vi "Scan Engine Initialization VI.vi"(8 "error in (no error)":errorcluster, 10 "Custom XML":string, 11 "Device Item Ref in":T1 format="%.0x") -> (0 "error out":errorcluster, 3 "Device Item Ref out":T1 format="%.0x")   [LabVIEW 2016, in "Scan Engine Custom Device.lvlib"]
uses:
  Scan Engine Custom Device.lvlib
  <vilib>/NI Veristand/Custom Device API/Custom Device Item Ref.ctl
  <vilib>/NI Veristand/Custom Device API/Custom Device Channel.ctl
  <vilib>/NI Veristand/Custom Device API/Custom Device Channel Type.ctl
  Globals/Property Strings.vi
  <vilib>/NI Veristand/Custom Device API/Set Item Property (U16).vi
  <vilib>/NI Veristand/Custom Device API/Set Item Property (String).vi
  <vilib>/NI Veristand/Custom Device API/Custom Device API.lvlib
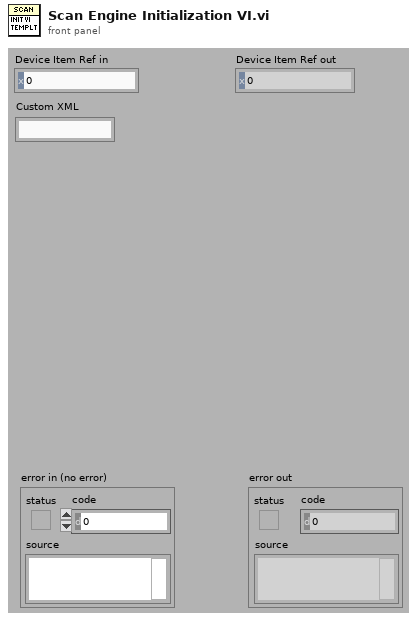
[diagram p1: front panel]
types:
  T1 = typedef "Custom Device API.lvlib/Custom Device Item Ref.ctl" = u64
  T2 = typedef "Custom Device API.lvlib/Custom Device Channel.ctl" = cluster{"Type":T3, "Units":string, "Default Value":dbl, "Faultable":bool, "Scalable":bool}
  T3 = typedef "Custom Device API.lvlib/Custom Device Channel Type.ctl" = enum16{"Input", "Output"}
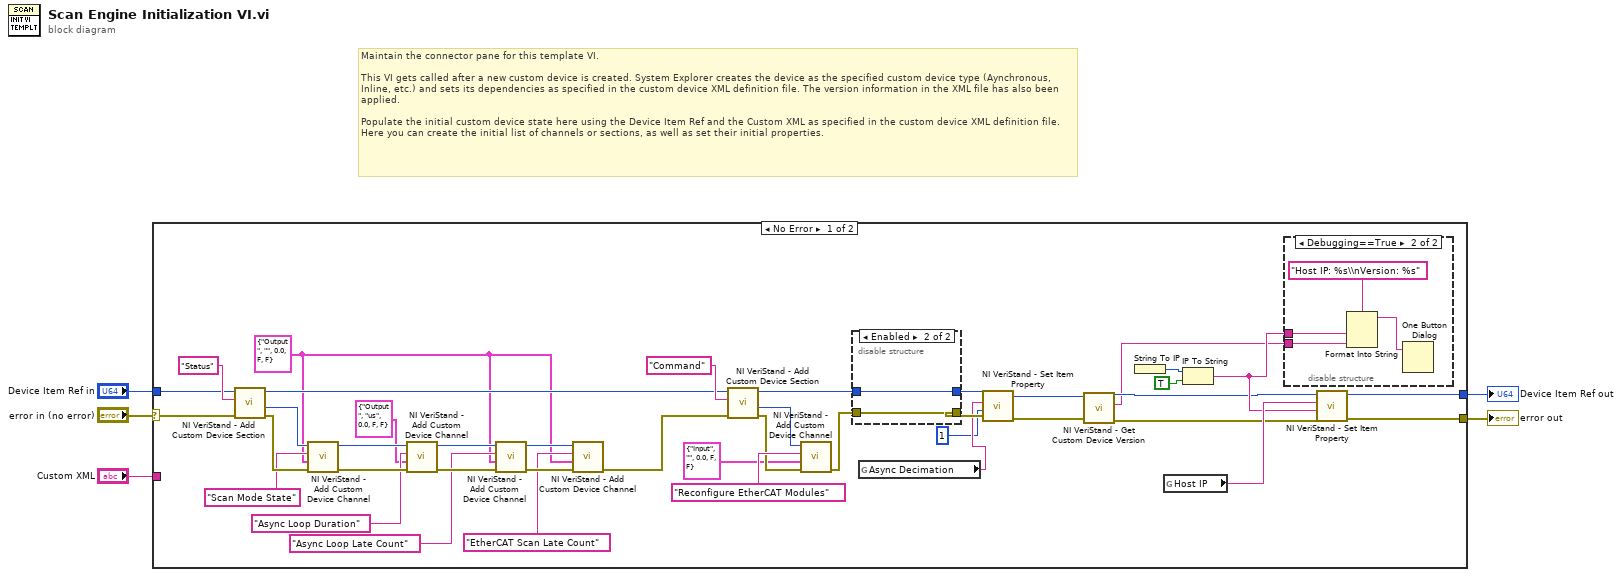
[diagram p0: block diagram]
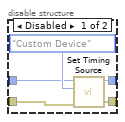
[diagram p3: hidden frame]
diagram:
  # "Maintain the connector pane for this template VI.\n\nThis VI gets called after a new custom device is created. System Explorer creates the device as the specified custom device type (Aynchronous, Inline, etc.) and sets its dependencies as specified in the custom device XML definition file. The version information in the XML file has also been applied.\n\nPopulate the initial custom device state here using the Device Item Ref and the Custom XML as specified in the custom device XML definition file. Here you can create the initial list of channels or sections, as well as set their initial properties."
  n1 = case shown="No Error" "error in (no error)" {
    selector: "error in (no error)" -> [w29 w59]
    tunnel: [w14 w59] -> w5
    tunnel: [w15 w58] -> w3
    tunnel: "Device Item Ref in" -> [w30 w58]
    tunnel: "Custom XML" -> [_ _]
    frame No Error {
      w17 = T2 {"Type"=enum."Output", "Units"="", "Default Value"=0.0, "Faultable"=FALSE, "Scalable"=FALSE} ("Channel")
      n2 = call <vilib>:"NI VeriStand - Add Custom Device Section.vi"("error in (no error)"=w29, "Section Name"="Status", "Parent Ref in"=w30) -> ("error out"=w44:errorcluster, "Section Ptr"=w45:T1, "Parent Ref out"=w37:T1)  [unwired: 5 in, 1 out]
      n3 = call <vilib>:"NI VeriStand - Add Custom Device Channel.vi"("error in (no error)"=w44, "Channel"=w17, "Channel Name"="Scan Mode State", "Parent Ref in"=w45) -> ("error out"=w28:errorcluster, "Parent Ref out"=w25:T1)  [unwired: 4 in, 2 out]
      n4 = call <vilib>:"NI VeriStand - Add Custom Device Channel.vi"("error in (no error)"=w28, "Channel"=T2 {"Type"=enum."Output", "Units"="us", "Default Value"=0.0, "Faultable"=FALSE, "Scalable"=FALSE}, "Channel Name"="Async Loop Duration", "Parent Ref in"=w25) -> ("error out"=w27:errorcluster, "Parent Ref out"=w26:T1)  [unwired: 4 in, 2 out]
      n5 = call <vilib>:"NI VeriStand - Add Custom Device Channel.vi"("error in (no error)"=w27, "Channel"=w17, "Channel Name"="Async Loop Late Count", "Parent Ref in"=w26) -> ("error out"=w21:errorcluster, "Parent Ref out"=w22:T1)  [unwired: 4 in, 2 out]
      n6 = call <vilib>:"NI VeriStand - Add Custom Device Channel.vi"("error in (no error)"=w21, "Channel"=w17, "Channel Name"="EtherCAT Scan Late Count", "Parent Ref in"=w22) -> ("error out"=w19:errorcluster)  [unwired: 4 in, 3 out]
      n7 = call <vilib>:"NI VeriStand - Add Custom Device Section.vi"("error in (no error)"=w19, "Section Name"="Command", "Parent Ref in"=w37) -> ("error out"=w41:errorcluster, "Section Ptr"=w40:T1, "Parent Ref out"=w36:T1)  [unwired: 5 in, 1 out]
      n8 = call <vilib>:"NI VeriStand - Add Custom Device Channel.vi"("error in (no error)"=w41, "Channel"=T2 {"Type"=enum."Input", "Units"="", "Default Value"=0.0, "Faultable"=FALSE, "Scalable"=FALSE}, "Channel Name"="Reconfigure EtherCAT Modules", "Parent Ref in"=w40) -> ("error out"=w35:errorcluster)  [unwired: 4 in, 3 out]
      n9 = disable-structure shown="Enabled" {
        disable-tunnel: w36 -> [w54 w57]
        disable-tunnel: w35 -> [w53 w56]
        disable-tunnel: [w52 w57] -> w34
        disable-tunnel: [w51 w56] -> w33
        frame Disabled {
          n10 = call "Set Timing Source.vi"("error in (no error)"=w53, "Timing Source"=enum16{"Automatic", "Custom Device"}."Custom Device", "Item Ref in"=w54) -> ("error out"=w51:errorcluster, "Item Ref out"=w52:T1)  [unwired: 7 in]
        }
        frame Enabled {
        }
      }
      n11 = global read "Property Strings.vi" "Async Decimation"() -> (w32:string)
      n12 = call-poly <vilib>:"NI VeriStand - Set Item Property.vi"("error in (no error)"=w33, "Value"=u16 1, "Property Name"=w32, "Item Ref in"=w34) -> ("error out"=w9:errorcluster, "Item Ref out"=w10:T1)  [unwired: 5 in, 1 out]
      n13 = call <vilib>:"NI VeriStand - Get Custom Device Version.vi"("error in (no error)"=w9, "Device Ref in"=w10) -> ("error out"=w8:errorcluster, "Value"=w6:string, "Device Ref out"=w7:T1)  [unwired: 7 in]
      n14 = String To IP() -> (0:w13:u32)  [unwired: 1 in]
      n15 = global read "Property Strings.vi" "Host IP"() -> (w16:string)
      n16 = IP To String(1:TRUE ("dot notation? (F)"), 2:w13) -> (0:w11:string)
      n17 = disable-structure shown="Debugging==True" {
        disable-tunnel: w11 -> [_ w50]
        disable-tunnel: w6 -> [_ w47]
        frame condition #0 {
        }
        frame condition #1 (active) {
          n18 = Format Into String(format string="Host IP: %s\\nVersion: %s", w50, w47) -> (resulting string=w49:string)  [unwired: 2 in, 1 out]
          n19 = One Button Dialog(message=w49) -> ()  [unwired: 1 in, 1 out]
        }
      }
      n20 = call-poly <vilib>:"NI VeriStand - Set Item Property.vi"("error in (no error)"=w8, "Value"=w11, "Property Name"=w16, "Item Ref in"=w7) -> ("error out"=w14:errorcluster, "Item Ref out"=w15:T1)  [unwired: 5 in, 1 out]
    }
    frame Error {
    }
  }
  "error out" <- w5
  "Device Item Ref out" <- w3
